vi "Add test result.vi"(10 "Test Result":T1, 11 "LUnit Test Case In":refnum<class "LUnit Test Case V2.lvclass">) -> (3 "LUnit Test Case Out":refnum<class "LUnit Test Case V2.lvclass">)   [LabVIEW 2020]
uses:
  LUnit Test Case V2.lvclass
  LUnit Test Case V2.lvclass/LUnit Test Case V2.ctl
  Framework/Result Types/Method Result/Public/Aggregate Assertion Results.vi
  Framework/Result Types/Method Result/Private/Merge Status.vi
  Framework/Result Types/Method Result/Private/Concatenate result strings.vi
  Framework/Result Types/Assertion Result/Public/TypeDefs/Status.ctl
  Framework/Result Types/Assertion Result/Assertion Result.lvlib
  Framework/Result Types/Assertion Result/Public/TypeDefs/Assertion Type.ctl
  Framework/Result Types/Assertion Result/Assertion Result.ctl
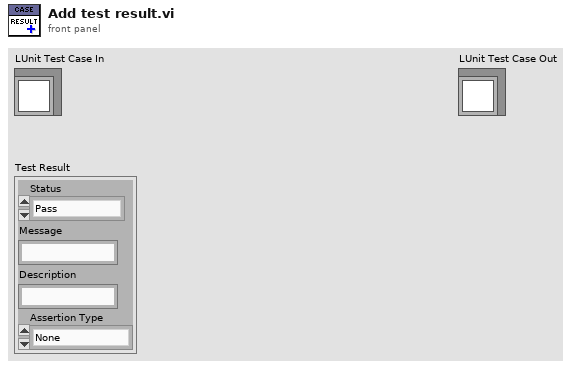
[diagram p1: front panel]
types:
  T1 = typedef "Assertion Result.lvlib/Assertion Result.ctl" = cluster{"Status":T2, "Message":string, "Description":string, "Assertion Type":T3}
  T2 = typedef "Assertion Result.lvlib/Status.ctl" = enum16{"Pass", "Fail", "Error", "Skipped", "Setup Error", "Broken", "Teardown Error"}
  T3 = typedef "Assertion Result.lvlib/Assertion Type.ctl" = enum16{"None", "Pass", "Fail", "Skip", "Pass if Equal", "Fail if Equal", "Pass if Error", "Fail if Error", "Pass if", "Fail if"}
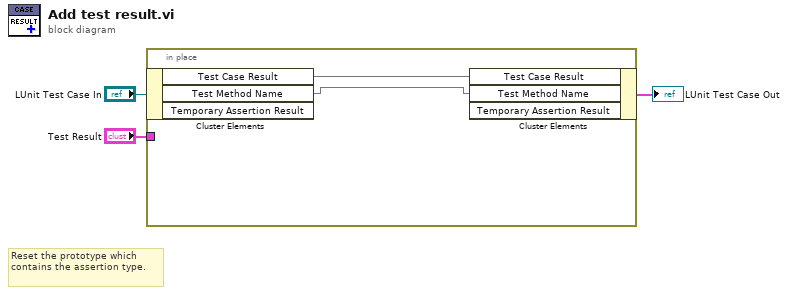
[diagram p0: block diagram]
diagram:
  # "Reset the prototype which contains the assertion type."
  n1 = in-place {
    in-place-border: "Test Result" -> [_]
    n2 = in-place-cluster #1("LUnit Test Case In") -> ("Test Case Result"=w6, "Test Method Name"=w5)  [unwired: 1 out]
    n3 = in-place-cluster #1("Test Case Result"=w6, "Test Method Name"=w5) -> (→"LUnit Test Case Out":cluster{}, "Temporary Assertion Result"=w4)
  }
